vi "getCurrentTone.vi"(8 "error in":errorcluster, 11 "signal":waveform(dbl)) -> (0 "error out":errorcluster, 2 "tone":i32, 3 "vaild?":bool)   [LabVIEW 2013]
uses:
  <vilib>/express/express analysis/Spectral/Block/exnSpectralBlock spectral measurements RMS poly.vi
  <vilib>/express/express analysis/Spectral/Block/exnSpectralBlock spectral measurements RMS DDT.vi
  <vilib>/Waveform/WDTOps.llb/WDT Get XY Value DBL.vi
  <vilib>/express/express analysis/Spectral/XNode/ExpressSpectralMeasurementsBlockNode.xnode
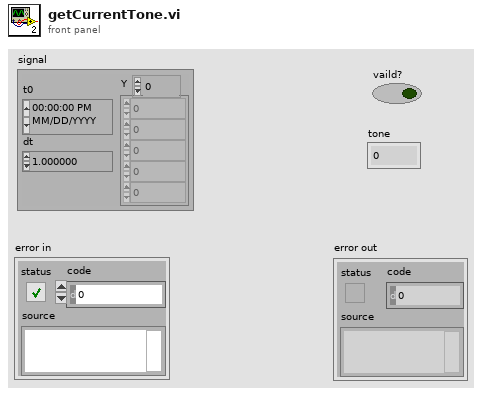
[diagram p1: front panel]
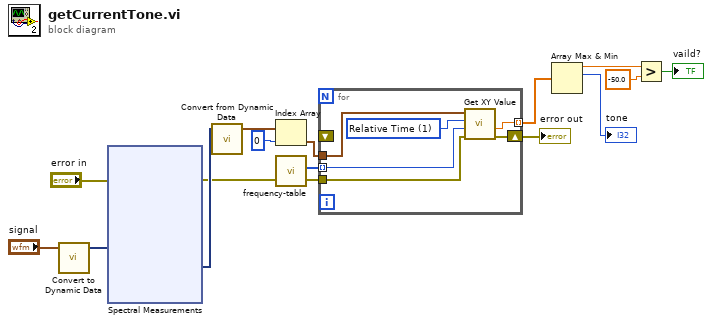
[diagram p0: block diagram]
diagram:
  n1 = call "Convert to Dynamic Data"("Waveform"="signal") -> ("Dynamic Data Type"=w5:dynamicdata)  [unwired: 3 in]
  n2 = xnode "Spectral Measurements"("Signals"=w5, "error in (no error)"="error in") -> ("FFT - (RMS)"=w15:dynamicdata, "error out"=w2:errorcluster)  [unwired: 1 out]
  n3 = call "Convert from Dynamic Data"("Dynamic Data Type"=w15) -> ("Array of Waveform"=w13:waveform(dbl)[])  [unwired: 3 in]
  n4 = Index Array(array=w13, index=0) -> (element=w11:waveform(dbl))
  n5 = call "frequency-table.vi"() -> ("value"=w14:i32[])  [unwired: 11 in]
  n6 = for {
    tunnel: w14 -> [w19] mode=indexing
    tunnel: [w18] -> w4 mode=indexing
    tunnel: w11 -> [w21]
    tunnel: w2 -> [w17]
    shift-right: [w16] -> w1
    shift-left: _ -> [_]
    w20 = u16 1 items=["Samples", "Relative Time"] ("Y position format")
    n7 = call-poly <vilib>:"Get XY Value.vi"("error in (no error)"=w17, "Y position"=w19, "Y position format"=w20, "waveform in"=w21) -> ("error out"=w16:errorcluster, "Y value"=w18:dbl)  [unwired: 3 in, 3 out]
  }
  "error out" <- w1
  n8 = Array Max & Min(array=w4) -> (max value=w10:dbl, max index (indices)=→"tone":i32)  [unwired: 2 out]
  n9 = Greater?(x=w10, y=-50.0) -> (0:→"vaild?":bool)
